vi "Omega CN9600 Simple Control.vi"() -> ()   [LabVIEW 2014]
uses:
  Omega/Serial_Config_Omega.ctl
  Omega/Omega CN9600 series.lvclass
  <vilib>/Utility/error.llb/DialogType.ctl
  <vilib>/ErrorRing/Error Ring.xnode
panel:
  out "error out":errorcluster
  in  "stop":bool
  in  "Connect":bool
  in  "Serial Config":T1={"Baud"=9600, "Flow Ctl"=0, "Parity"=0, "Address"=1, "VISA resource name"="COM5"} {"Parity" items=["None", "Odd", "Even"]; "Flow Ctl" items=["None"]; "Baud" items=["4800"=4800, "9600"=9600, "19200"=19200, "38400"=38400]}
  in  "Setpoint":dbl format="%.1f"
  out "Temperature":dbl format="%.1f"
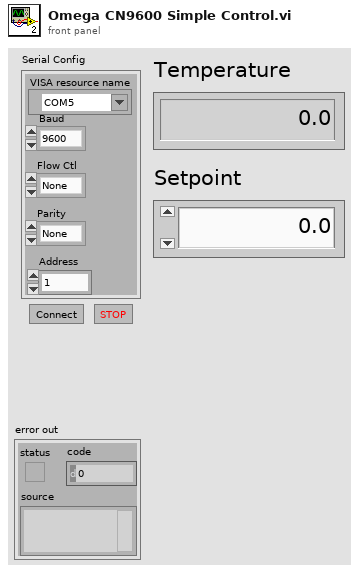
[diagram p1: front panel]
types:
  T1 = typedef "Omega CN9600 series.lvclass/Serial_Config_Omega.ctl" = cluster{"Baud":u32, "Flow Ctl":u16, "Parity":u16, "Address":u8, "VISA resource name":refnum<visa-resource-name>}
  T2 = enum32{"invalid app kind", "Development System", "Run Time System", "Student Edition", "Embedded LabVIEW", "Evaluation", "Custom"}
  T3 = typedef "DialogType.ctl" = u16
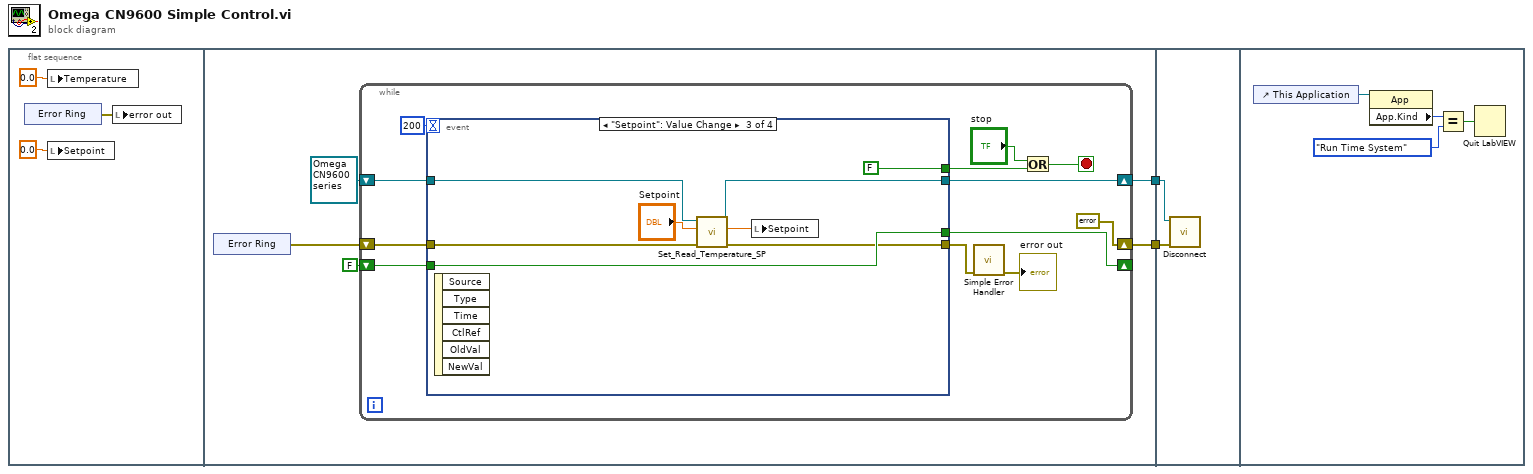
[diagram p0: block diagram]
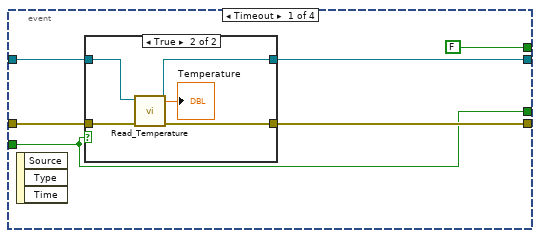
[diagram p2: hidden frame]
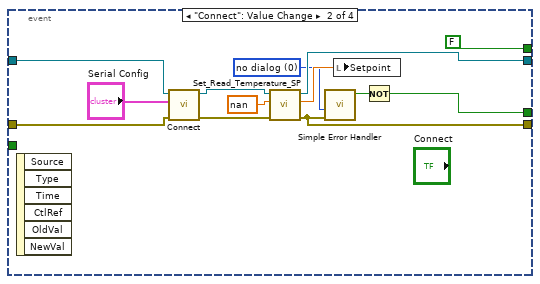
[diagram p4: hidden frame]
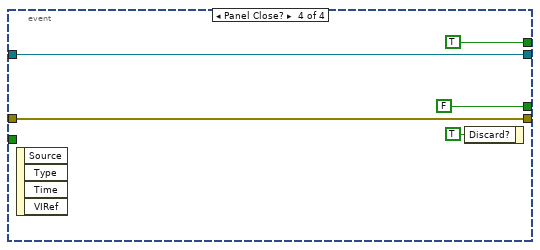
[diagram p5: hidden frame]
diagram:
  n1 = flat-sequence {
    tunnel: [w8] -> w2
    tunnel: [w7] -> w1
    tunnel: w2 -> [w65]
    tunnel: w1 -> [w64]
    frame #0 {
      n2 = xnode "Error Ring"() -> ("error out"=w3:errorcluster)
      n3 = local write "Temperature"(0.0 ("Temperature")) -> ()
      n4 = local write "Setpoint"(0.0 ("Setpoint")) -> ()
      n5 = local write "error out"(w3) -> ()
    }
    frame #1 {
      n6 = xnode "Error Ring"() -> ("error out"=w11:errorcluster)
      n7 = while {
        shift-right: [w21] -> w8
        shift-left: refnum<class "Omega CN9600 series.lvclass"> refnum ("Omega CN9600 series.lvclass") -> [w23]
        shift-right: [errorcluster {"status"=FALSE, "code"=0, "source"=""} ("error out")] -> w7
        shift-left: w11 -> [w22]
        shift-right: [w19] -> _
        shift-left: FALSE -> [w20]
        stop <- w13 stop-if-true
        n8 = event shown="[2] \"Setpoint\": Value Change" {
          selector: _ -> [_ _ _ _]
          dyn-events: _ -> [_ _ _ _]
          timeout: 200 -> [_ _ _ _]
          tunnel: w23 -> [w30 w50 w58 w63]
          tunnel: w22 -> [w29 w49 w56 w59]
          tunnel: [w28 w47 w53 w63] -> w21
          tunnel: [w27 w41 w54 w59] -> w17
          tunnel: w20 -> [w26 _ w55 _]
          tunnel: [w26 w39 w55 FALSE] -> w19
          tunnel: [FALSE ("stop") FALSE ("stop") FALSE ("stop") TRUE ("stop")] -> w14
          event Timeout {
            n9 = event-data() -> ()  [unwired: 1 in, 3 out]
            n10 = case shown="True" w26 {
              tunnel: w30 -> [w32 w37]
              tunnel: w29 -> [w31 w36]
              tunnel: [w32 w35] -> w28
              tunnel: [w31 w33] -> w27
              frame False {
              }
              frame True {
                n11 = call "Read_Temperature.vi"("error in (no error)"=w36, "Omega CN9600 series.lvclass"=w37) -> ("error out"=w33:errorcluster, "Temperature"=→"Temperature":dbl, "Omega CN9600 series.lvclass 2"=w35:refnum<class "Omega CN9600 series.lvclass">)  [unwired: 7 in]
              }
            }
          }
          event "Connect": Value Change {
            w40 = T3 0 items=["no dialog", "OK message", "continue or stop message", "OK message + warnings", "continue/stop + warnings"] ("type of dialog (OK msg:1)")
            n12 = event-data() -> ()  [unwired: 1 in, 6 out]
            n13 = call "Connect.vi"("error in (no error)"=w49, "Serial Config"="Serial Config", "Omega CN9600 series.lvclass"=w50) -> ("error out"=w46:errorcluster, "Omega CN9600 series.lvclass 2"=w48:refnum<class "Omega CN9600 series.lvclass">)  [unwired: 7 in]
            n14 = call "Set_Read_Temperature_SP.vi"("error in (no error)"=w46, "setpoint"=nan, "Omega CN9600 series.lvclass"=w48) -> ("error out"=w41:errorcluster, "actual setpoint"=w45:dbl, "Omega CN9600 series.lvclass 2"=w47:refnum<class "Omega CN9600 series.lvclass">)  [unwired: 5 in]
            n15 = call <vilib>:"Simple Error Handler.vi"("type of dialog (OK msg:1)"=w40, "error in (no error)"=w41) -> ("error?"=w38:bool)  [unwired: 3 in, 4 out]
            n16 = local write "Setpoint"(w45) -> ()
            n17 = Not(x=w38) -> (.not. x?=w39:bool)
          }
          event "Setpoint": Value Change {
            n18 = event-data() -> ()  [unwired: 1 in, 6 out]
            n19 = call "Set_Read_Temperature_SP.vi"("error in (no error)"=w56, "setpoint"="Setpoint", "Omega CN9600 series.lvclass"=w58) -> ("error out"=w54:errorcluster, "actual setpoint"=w52:dbl, "Omega CN9600 series.lvclass 2"=w53:refnum<class "Omega CN9600 series.lvclass">)  [unwired: 5 in]
            n20 = local write "Setpoint"(w52) -> ()
          }
          event Panel Close? {
            n21 = event-data() -> ()  [unwired: 1 in, 4 out]
            n22 = event-data("Discard?"=TRUE) -> ()  [unwired: 1 in, 1 out]
          }
        }
        n23 = call <vilib>:"Simple Error Handler.vi"("error in (no error)"=w17) -> ("error out"=→"error out":errorcluster)  [unwired: 4 in, 4 out]
        n24 = Or(x="stop", y=w14) -> (x .or. y?=w13:bool)
      }
    }
    frame #2 {
      n25 = call "Disconnect.vi"("error in (no error)"=w64, "Omega CN9600 series.lvclass"=w65) -> ()  [unwired: 9 in, 1 out]
    }
    frame #3 {
      n26 = control-ref of="This Application"() -> (w69:refnum<vi>)
      n27 = property class="App"(reference=w69) -> ("App.Kind"=w68:T2)  [unwired: 1 in, 2 out]
      n28 = Equal?(x=w68, y=T2."Run Time System") -> (x = y?=w66:bool)
      n29 = Quit LabVIEW(quit? (T)=w66) -> ()
    }
  }
